vi "Cluster to Meta Data.vi"(8 "error in":errorcluster, 11 "Configuration Cluster":variant) -> (0 "error out":errorcluster, 3 "configuration_parameters":T1(array[cluster]))   [LabVIEW 2020, in "LoadRegulation.lvlib" / "MeasurementService_Template.lvclass"]
uses:
  MeasurementService_Template.lvclass
  <vilib>/Utility/Data Type/NI_Data Type.lvlib
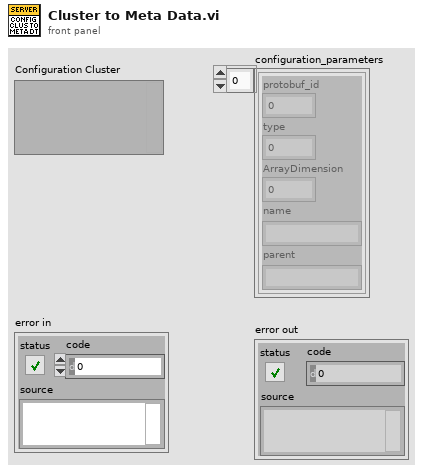
[diagram p1: front panel]
types:
  T1 = cluster{"protobuf_id":i32, "type":i32, "ArrayDimension":i32, "name":string, "parent":string}[]
  T2 = typedef "NI_Data Type.lvlib/Data Type.ctl" = enum8{"Invalid Type", "Void", "I8", "I16", "I32", "I64", "U8", "U16", "U32", "U64", "Single Float", "Double Float", "Extended Float", "Single Complex", "Double Complex", "Extended Complex", "Enum U8", "Enum U16", "Enum U32", "Enum U64", "Single Float With Unit", "Double Float With Unit", "Extended Float With Unit", "Single Complex with Unit", "Double Complex with Unit", "Extended Complex with Unit", "Boolean", "String", "Path", "Picture", "Tag", "Array", "Cluster", "Variant", "LV Variant", "Waveform", "Timestamp", "Digital Waveform", "Digital Data", "ExpressData", "Refnum", "External Data", "VI", "Poly VI", "LabVIEW Class Instance", "Fixed Point", "Set Collection", "Map Collection"}
  T3 = cluster{"protobuf_id":i32, "type":i32, "ArrayDimension":i32, "name":string, "parent":string}
  T4 = typedef "LoadRegulation.lvlib/MeasurementService_Template.lvclass/Measurement DataType.ctl" = enum16{"UNSPECIFIED", "BOOL", "DOUBLE", "FLOAT", "INT32", "INT64", "STRING", "UINT32", "UINT64"}
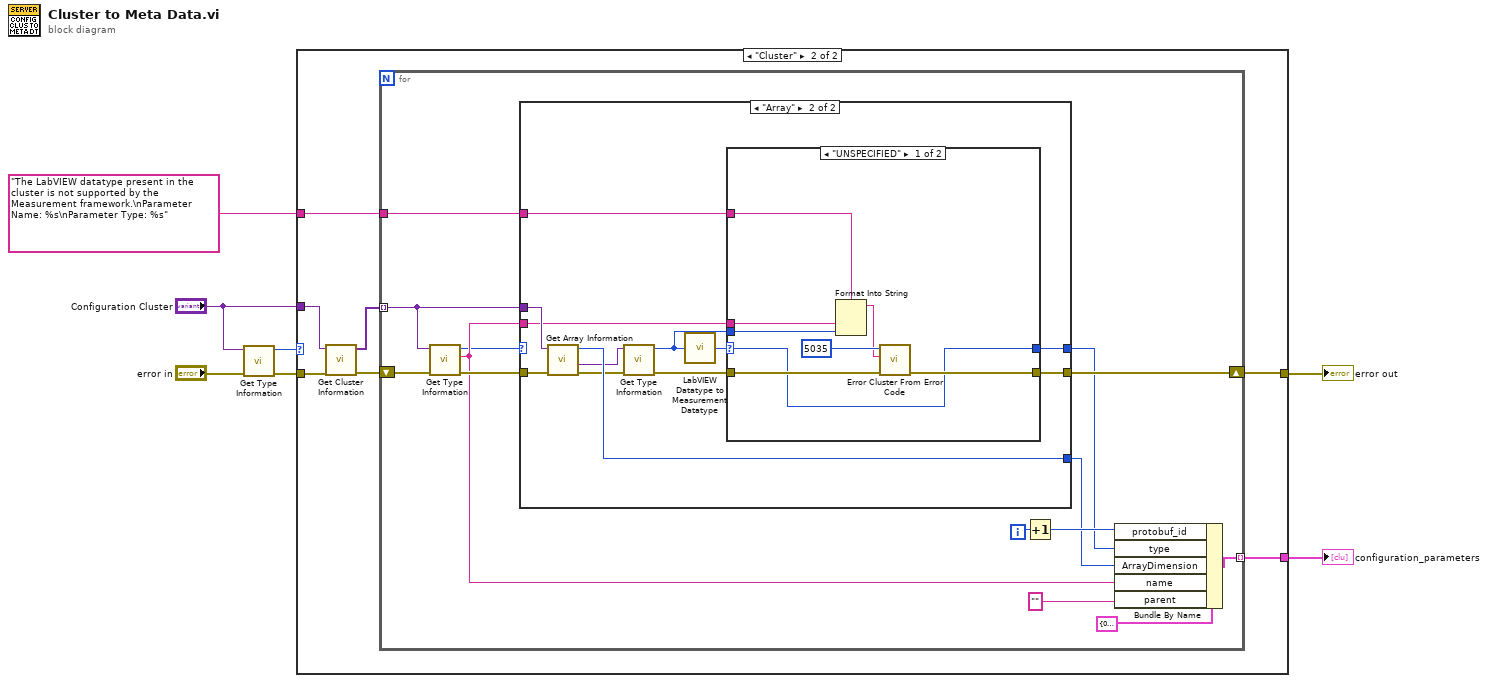
[diagram p0: block diagram]
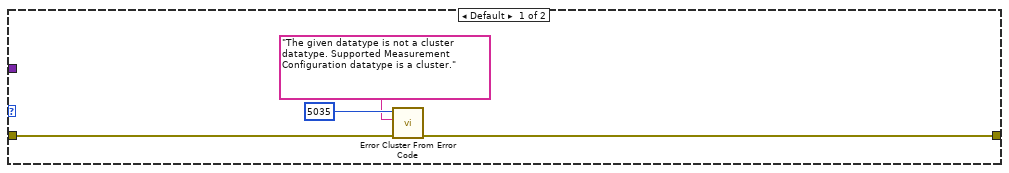
[diagram p2: hidden frame]
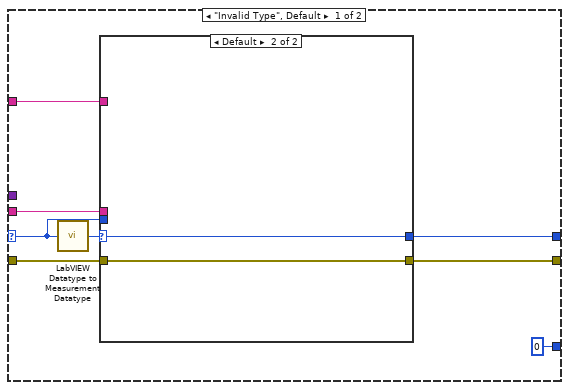
[diagram p3: hidden frame]
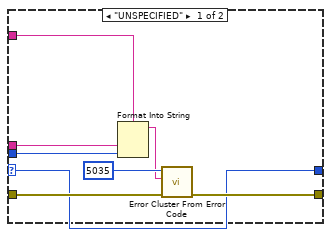
[diagram p4: hidden frame]
diagram:
  n1 = call <vilib>:"Get Type Information.vi"("error in (no error)"="error in", "variant"="Configuration Cluster") -> ("error out"=w6:errorcluster, "type"=w5:T2)  [unwired: 5 in, 3 out]
  n2 = case shown="\"Cluster\"" w5 {
    tunnel: w6 -> [w11 w18]
    tunnel: [w10 w13] -> w4
    tunnel: "Configuration Cluster" -> [_ w17]
    tunnel: [_ w14] -> w2
    tunnel: "The LabVIEW datatype present in the cluster is not supported by the Measurement framework.\nParameter Name: %s\nParameter Type: %s" ("error message (\"\")") -> [_ w12]
    frame Default {
      n3 = call <vilib>:"Error Cluster From Error Code.vi"("error in (no error)"=w11, "error message (\"\")"="The given datatype is not a cluster datatype. Supported Measurement Configuration datatype is a cluster." ("error message (\"\")"), "error code (0)"=5035) -> ("error out"=w10:errorcluster)  [unwired: 6 in]
    }
    frame "Cluster" {
      n4 = call <vilib>:"Get Cluster Information.vi"("error in (no error)"=w18, "variant"=w17) -> ("error out"=w16:errorcluster, "cluster elements"=w15:variant[])  [unwired: 8 in]
      n5 = for {
        tunnel: w15 -> [w22] mode=indexing
        tunnel: [w30] -> w14 mode=indexing
        shift-right: [w28] -> w13
        shift-left: w16 -> [w32]
        tunnel: w12 -> [w19]
        i -> [w24]
        n6 = call <vilib>:"Get Type Information.vi"("error in (no error)"=w32, "variant"=w22) -> ("error out"=w29:errorcluster, "name"=w27:string, "type"=w26:T2)  [unwired: 5 in, 2 out]
        n7 = case shown="\"Array\"" w26 {
          selector: w26 -> [w36 _]
          tunnel: w29 -> [w39 w62]
          tunnel: [w38 w52] -> w28
          tunnel: w27 -> [w37 w54]
          tunnel: w22 -> [_ w61]
          tunnel: [w35 w53] -> w21
          tunnel: [0 ("number of dimensions") w60] -> w20
          tunnel: w19 -> [w33 w51]
          frame "Invalid Type", Default {
            n8 = call "LabVIEW Datatype to Measurement Datatype.vi"("LabVIEW type"=w36) -> ("Measurement DataType"=w40:T4)
            n9 = case shown="Default" w40 {
              selector: w40 -> [w42 w49]
              tunnel: w39 -> [w47 w50]
              tunnel: [w46 w50] -> w38
              tunnel: w37 -> [w44 _]
              tunnel: w36 -> [w43 _]
              tunnel: [w42 w49] -> w35
              tunnel: w33 -> [w41 _]
              frame "UNSPECIFIED" {
                n10 = Format Into String(format string=w41, w44, w43) -> (resulting string=w45:string)  [unwired: 2 in, 1 out]
                n11 = call <vilib>:"Error Cluster From Error Code.vi"("error in (no error)"=w47, "error message (\"\")"=w45, "error code (0)"=5035) -> ("error out"=w46:errorcluster)  [unwired: 6 in]
              }
              frame Default {
              }
            }
          }
          frame "Array" {
            n12 = call <vilib>:"Get Array Information.vi"("error in (no error)"=w62, "variant"=w61) -> ("error out"=w59:errorcluster, "array element data type"=w55:variant, "number of dimensions"=w60:i32)  [unwired: 6 in, 1 out]
            n13 = call <vilib>:"Get Type Information.vi"("error in (no error)"=w59, "variant"=w55) -> ("error out"=w57:errorcluster, "type"=w56:T2)  [unwired: 5 in, 3 out]
            n14 = call "LabVIEW Datatype to Measurement Datatype.vi"("LabVIEW type"=w56) -> ("Measurement DataType"=w58:T4)
            n15 = case shown="\"UNSPECIFIED\"" w58 {
              selector: w58 -> [w64 w71]
              tunnel: w57 -> [w69 w72]
              tunnel: [w68 w72] -> w52
              tunnel: w54 -> [w66 _]
              tunnel: w56 -> [w65 _]
              tunnel: [w64 w71] -> w53
              tunnel: w51 -> [w63 _]
              frame "UNSPECIFIED" {
                n16 = Format Into String(format string=w63, w66, w65) -> (resulting string=w67:string)  [unwired: 2 in, 1 out]
                n17 = call <vilib>:"Error Cluster From Error Code.vi"("error in (no error)"=w69, "error message (\"\")"=w67, "error code (0)"=5035) -> ("error out"=w68:errorcluster)  [unwired: 6 in]
              }
              frame Default {
              }
            }
          }
        }
        n18 = Increment(x=w24) -> (x+1=w23:i32)
        n19 = Bundle By Name(cluster=T3 {"protobuf_id"=0, "type"=0, "ArrayDimension"=0, "name"="", "parent"=""} ("Measurement_v1_ConfigurationParameter_Data"), "protobuf_id"=w23, "type"=w21, "ArrayDimension"=w20, "name"=w27, "parent"="") -> (w30:T3)
      }
    }
  }
  "error out" <- w4
  "configuration_parameters" <- w2
